vi "CloseOneGraph.vi"(8 "error in (no error)":errorcluster, 9 "Graph name":string, 11 "Gserver in":refnum<class "Gserver.lvclass">) -> (0 "error out":errorcluster, 3 "Gserver out":refnum<class "Gserver.lvclass">)   [LabVIEW 2020, in "Sgraph_lib_V1.lvlib" / "Gserver.lvclass"]
doc: "Andre Koelewijn, 5 jan 2021\n\nSearch one Vserver Graph and send a close command.\nAlso remove the Graph Queue from Gserver Stack"
uses:
  Gserver.lvclass
  Gserver.lvclass/Gserver.ctl
  Gview/controls/Typedef_Gserver-Replies.ctl
  Gview/controls/Typedef_ServerActions.ctl
  Builds/Sgraph_lib_V1.lvlib
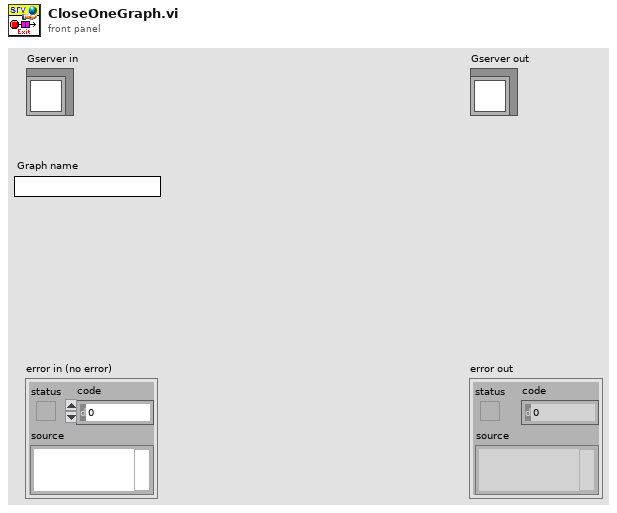
[diagram p1: front panel]
types:
  T1 = typedef "Sgraph_lib_V1.lvlib/Typedef_ServerActions.ctl" = enum16{"GraphUpdate", "SendAllTags", "SendIniPath", "SetGeneralOptions", "EditTagsOpen", "EditTagsPresetSave", "EditTagsPresetLoad", "EditTagsClose", "NewTagSelection", "ExitGraph"}
  T2 = typedef "Typedef_Gserver-Replies.ctl" = cluster{"ServerActions":T1, "data":variant, "Source":string, "Time Stamp":timestamp}
  T3 = typedef "Sgraph_lib_V1.lvlib/Gserver.lvclass/Typedef_PeriodicUpdate.ctl" = cluster{"Sending Gviewer":string, "PreviousUpdate":timestamp, "UpdateRate":dbl, "DataRequest":T4}
  T4 = typedef "Sgraph_lib_V1.lvlib/Gviewer.lvclass/Typedef_datarequest.ctl" = cluster{"Tags":string[], "Live":T5, "Time-Start":timestamp, "Time-End":timestamp, "TimeSpan":dbl, "DisplayResolution":i32}
  T5 = typedef "Sgraph_lib_V1.lvlib/Gviewer.lvclass/Typedef_Live.ctl" = enum16{"Live View", "Freeze"}
  T6 = typedef "Sgraph_lib_V1.lvlib/Gserver.lvclass/Typedef_Sgraph_Query.ctl" = cluster{"ViewportName":string, "Tags":string[], "Time-Start":timestamp, "Time-End":timestamp, "Pixels":i32, "Live":T5, "TimeSpan(sec)":dbl, "GViewer-Queue":refnum<queue>}
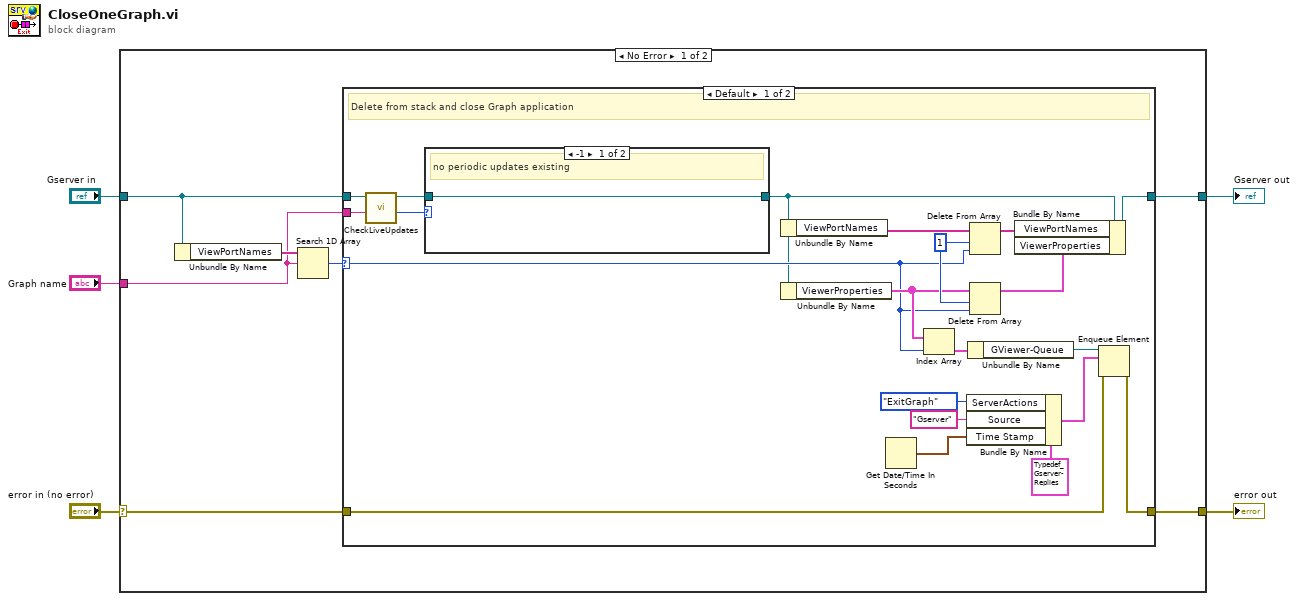
[diagram p0: block diagram]
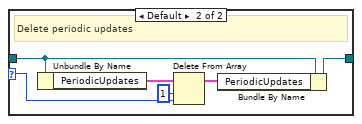
[diagram p2: hidden frame]
diagram:
  n1 = case shown="No Error" "error in (no error)" {
    selector: "error in (no error)" -> [w10 w44]
    tunnel: [w9 w44] -> w4
    tunnel: [w8 w43] -> w2
    tunnel: "Gserver in" -> [w7 w43]
    tunnel: "Graph name" -> [w6 _]
    frame No Error {
      n2 = Unbundle By Name(w7) -> ("ViewPortNames"=w12:string[])
      n3 = Search 1D Array(1D array=w12, element=w6) -> (index of element=w11:i32)  [unwired: 1 in]
      n4 = case shown="Default" w11 {
        selector: w11 -> [w28 _]
        tunnel: w7 -> [w17 w42]
        tunnel: [w18 w42] -> w8
        tunnel: w10 -> [w21 w41]
        tunnel: [w20 w41] -> w9
        tunnel: w6 -> [w16 _]
        frame Default {
          w30 = 1 ("length")
          # "Delete from stack and close Graph application"
          n5 = call "CheckLiveUpdates.vi"("GraphName"=w16, "Gserver in"=w17) -> ("index"=w15:i32, "Gserver out"=w14:refnum<class "Gserver.lvclass">)  [unwired: 7 in, 1 out]
          n6 = case shown="-1" w15 {
            selector: w15 -> [_ w38]
            tunnel: w14 -> [w34 w35]
            tunnel: [w34 w36] -> w13
            frame -1 {
              # "no periodic updates existing"
            }
            frame Default {
              # "Delete periodic updates"
              n7 = Unbundle By Name(w35) -> ("PeriodicUpdates"=w40:T3[])
              n8 = Delete From Array(array=w40, length=1, index=w38) -> (array with subset deleted=w37:T3[])  [unwired: 1 out]
              n9 = Bundle By Name(cluster=w35, "PeriodicUpdates"=w37) -> (w36:refnum<class "Gserver.lvclass">)
            }
          }
          n10 = Unbundle By Name(w13) -> ("ViewPortNames"=w33:string[])
          n11 = Unbundle By Name(w13) -> ("ViewerProperties"=w29:T6[])
          n12 = Get Date/Time In Seconds() -> (seconds since 1Jan1904=w26:timestamp)
          n13 = Index Array(array=w29, index=w28) -> (element=w24:T6)
          n14 = Bundle By Name(cluster=T2 {"ServerActions"=enum."GraphUpdate", "data"=variant, "Source"="", "Time Stamp"=timestamp(0 s since 1904-01-01)} ("element"), "ServerActions"=Typedef_ServerActions."ExitGraph", "Source"="Gserver", "Time Stamp"=w26) -> (w22:T2)
          n15 = Unbundle By Name(w24) -> ("GViewer-Queue"=w27:refnum<queue>)
          n16 = Delete From Array(array=w33, length=w30, index=w28) -> (array with subset deleted=w32:string[])  [unwired: 1 out]
          n17 = Delete From Array(array=w29, length=w30, index=w28) -> (array with subset deleted=w31:T6[])  [unwired: 1 out]
          n18 = Bundle By Name(cluster=w13, "ViewPortNames"=w32, "ViewerProperties"=w31) -> (w18:refnum<class "Gserver.lvclass">)
          n19 = Enqueue Element(queue=w27, element=w22, error in (no error)=w21) -> (error out=w20:errorcluster)  [unwired: 1 in, 2 out]
        }
        frame -1 {
          # "Viewport Graph not found"
        }
      }
    }
    frame Error {
    }
  }
  "error out" <- w4
  "Gserver out" <- w2
